vi "process(Client).vi"(8 "error in (no error)":errorcluster, 10 "Sync":refnum<notifier>, 11 "Session in":refnum<class "Session.lvclass">) -> (0 "error out":errorcluster, 3 "Session out":refnum<class "Session.lvclass">)   [LabVIEW 2013, in "MQTT Server.lvlib" / "Session.lvclass"]
uses:
  Session.lvclass
  Control Packets/ControlPacket/ControlPacket.lvclass
  Session.lvclass/Session.ctl
  Connection/TCPConnection.lvclass
panel:
  out "Last Packet":timestamp
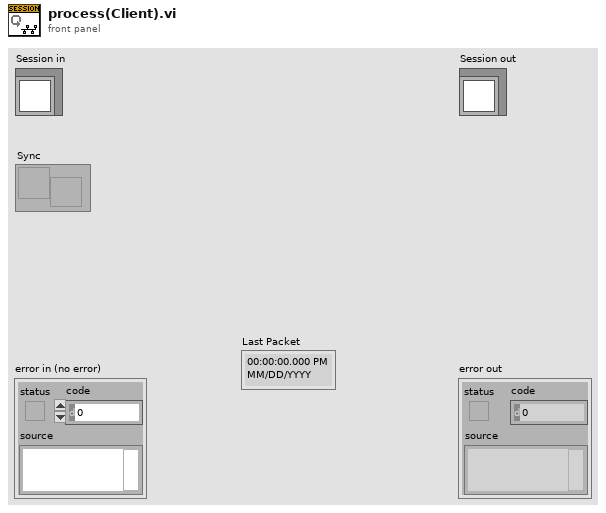
[diagram p1: front panel]
types:
  T1 = enum16{"Standard", "Buffered", "CRLF", "Immediate"}
  T2 = typedef "MQTT Server.lvlib/MQTT_Base.lvclass/Response -- cluster.ctl" = cluster{"Packet":refnum<class "ControlPacket.lvclass">, "Protocol Error":errorcluster, "disconnect session":bool}
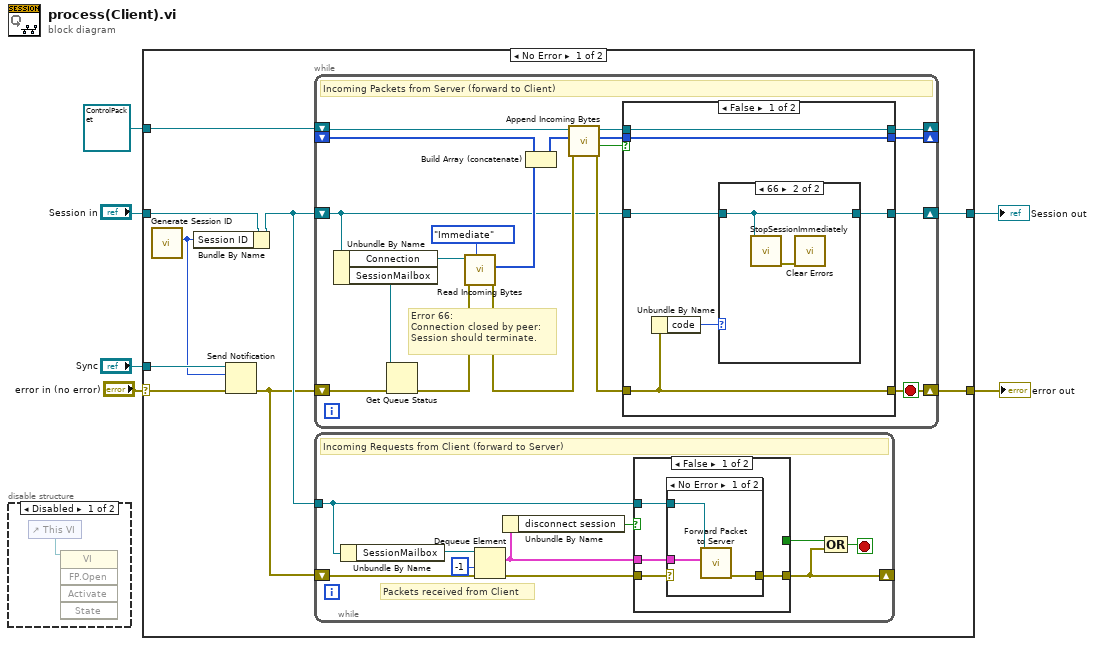
[diagram p0: block diagram]
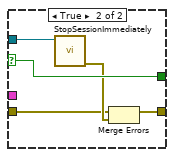
[diagram p4: hidden frame]
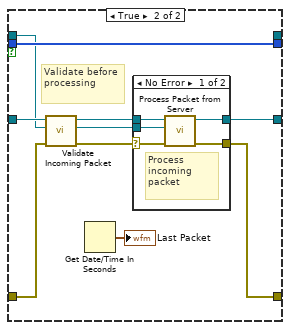
[diagram p6: hidden frame]
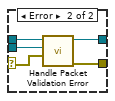
[diagram p7: hidden frame]
diagram:
  n1 = disable-structure shown="Disabled" {
    frame Disabled {
      n2 = control-ref of="This VI"() -> (w7:refnum<vi>)
      n3 = invoke class="VI" method="FP.Open"(reference=w7) -> ()  [unwired: 4 in, 5 out]
    }
    frame Enabled {
    }
  }
  n4 = case shown="No Error" "error in (no error)" {
    selector: "error in (no error)" -> [w12 w89]
    tunnel: [w8 w89] -> w3
    tunnel: [w13 w88] -> w2
    tunnel: "Session in" -> [w16 w88]
    tunnel: refnum<class "ControlPacket.lvclass"> refnum ("Incomplete ControlPacket") -> [w9 _]
    tunnel: "Sync" -> [w15 _]
    frame No Error {
      n5 = call "Generate Session ID.vi"() -> ("Session ID"=w10:i32)  [unwired: 11 in]
      n6 = Bundle By Name(cluster=w16, "Session ID"=w10) -> (w14:refnum<class "Session.lvclass">)
      n7 = Send Notification(notification=w10, notifier=w15, error in (no error)=w12) -> (error out=w11:errorcluster)  [unwired: 1 out]
      n8 = while {
        shift-right: [w48] -> w13
        shift-left: w14 -> [w40]
        shift-right: [w42] -> w8
        shift-left: w11 -> [w45]
        shift-right: [w54] -> _
        shift-left: w9 -> [w58]
        shift-right: [w52] -> _
        shift-left: _ -> [w51]
        stop <- w42 stop-if-true
        # "Error 66: \nConnection closed by peer:\nSession should terminate."
        # "Incoming Packets from Server (forward to Client)"
        n9 = Unbundle By Name(w40) -> ("Connection"=w57:refnum<class "TCPConnection.lvclass">, "SessionMailbox"=w46:refnum<queue>)
        n10 = Get Queue Status(queue=w46, error in (no error)=w45) -> (error out=w44:errorcluster)  [unwired: 1 in, 7 out]
        n11 = call "Read Incoming Bytes.vi"("mode (standard)"=T1."Immediate", "error in (no error)"=w44, "TCPConnection in"=w57) -> ("error out"=w47:errorcluster, "Bytes"=w50:u8[])  [unwired: 5 in, 2 out]
        n12 = Build Array (concatenate)(w51, w50) -> (w49:u8[])
        n13 = call "Append Incoming Bytes.vi"("error in (no error)"=w47, "Incoming Packets"=w49, "Incomplete ControlPacket"=w58) -> ("error out"=w41:errorcluster, "Complete Packet"=w56:bool, "Remaining Packets"=w53:u8[], "ControlPacket"=w55:refnum<class "ControlPacket.lvclass">)  [unwired: 5 in]
        n14 = case shown="False" w56 {
          tunnel: w55 -> [w64 w73]
          tunnel: [w64 _] -> w54
          tunnel: w53 -> [w63 w76]
          tunnel: [w63 w76] -> w52
          tunnel: [w60 w75] -> w48
          tunnel: w40 -> [w61 w74]
          tunnel: [w62 w68] -> w42
          tunnel: w41 -> [w62 w69]
          frame False {
            n15 = Unbundle By Name(w62) -> ("code"=w59:i32)
            n16 = case shown="66" w59 {
              tunnel: w61 -> [w65 w67]
              tunnel: [w65 w67] -> w60
              frame Default {
              }
              frame 66 {
                n17 = call "StopSessionImmediately.vi"("Session in"=w67) -> ("error out"=w66:errorcluster)  [unwired: 9 in, 1 out]
                n18 = call <vilib>:"Clear Errors.vi"("error in (no error)"=w66) -> ()  [unwired: 6 in, 1 out]
              }
            }
          }
          frame True {
            # "Validate before processing"
            n19 = call "Validate Incoming Packet.vi"("error in (no error)"=w69, "ControlPacket"=w73, "Session in"=w74) -> ("error out"=w70:errorcluster, "ControlPacket out"=w71:refnum<class "ControlPacket.lvclass">, "Session out"=w72:refnum<class "Session.lvclass">)  [unwired: 6 in]
            n20 = Get Date/Time In Seconds() -> (seconds since 1Jan1904=→"Last Packet":timestamp)
            n21 = case shown="No Error" w70 {
              selector: w70 -> [w80 w85]
              tunnel: [w79 w83] -> w75
              tunnel: w72 -> [w82 w87]
              tunnel: w71 -> [w81 w86]
              tunnel: [w78 w84] -> w68
              frame No Error {
                # "Process incoming packet"
                n22 = call "Process Packet from Server.vi"("error in (no error)"=w80, "Incoming Packet"=w81, "Session in"=w82) -> ("error out"=w78:errorcluster, "Session out"=w79:refnum<class "Session.lvclass">)  [unwired: 7 in]
              }
              frame Error {
                n23 = call "Handle Packet Validation Error.vi"("Packet Validation Error"=w85, "ControlPacket"=w86, "Session in"=w87) -> ("error out"=w84:errorcluster, "Session out"=w83:refnum<class "Session.lvclass">)  [unwired: 7 in]
              }
            }
          }
        }
      }
      n24 = while {
        tunnel: w14 -> [w22]
        shift-right: [w19] -> _
        shift-left: w11 -> [w23]
        stop <- w18 stop-if-true
        # "Packets received from Client"
        # "Incoming Requests from Client (forward to Server)"
        n25 = Unbundle By Name(w22) -> ("SessionMailbox"=w26:refnum<queue>)
        n26 = Dequeue Element(queue=w26, timeout in ms (-1)=-1, error in (no error)=w23) -> (element=w21:T2, error out=w24:errorcluster)  [unwired: 2 out]
        n27 = Unbundle By Name(w21) -> ("disconnect session"=w20:bool)
        n28 = case shown="False" w20 {
          selector: w20 -> [_ w39]
          tunnel: w24 -> [w30 w36]
          tunnel: [w29 w35] -> w19
          tunnel: w22 -> [w28 w38]
          tunnel: w21 -> [w27 _]
          tunnel: [_ w39] -> w17
          frame False {
            n29 = case shown="No Error" w30 {
              selector: w30 -> [_ w34]
              tunnel: w27 -> [w32 _]
              tunnel: [w31 w34] -> w29
              tunnel: w28 -> [w33 _]
              frame No Error {
                n30 = call "Forward Packet to Server.vi"("Message"=w32, "Session in"=w33) -> ("error out"=w31:errorcluster)  [unwired: 9 in]
              }
              frame Error {
              }
            }
          }
          frame True {
            n31 = call "StopSessionImmediately.vi"("Session in"=w38) -> ("error out"=w37:errorcluster)  [unwired: 9 in, 1 out]
            n32 = Merge Errors(w36, w37) -> (w35:errorcluster)
          }
        }
        n33 = Compound Arithmetic op=OR(w17, w19) -> (w18:bool)
      }
    }
    frame Error {
    }
  }
  "error out" <- w3
  "Session out" <- w2
